vi "load_manual.vi"(8 "error in (no error)":errorcluster) -> (0 "error out":errorcluster, 2 "replaced_action(s)":bool, 3 "manual_actions out":variant)   [LabVIEW 2015, in "lv-recipe-machine.lvlib" / "example_01.lvlib"]
doc: "load_manual.vi will assign manual steps as variant attributes to an empty variant. An indicator is provided if actions are replaced (e.g. a duplicate key)."
uses:
  example_01.lvlib
  public/_controls/step.ctl
  public/_controls/vi_reference_type.ctl
  _controls/steps_actions.ctl
  public/_controls/vi_reference_manual_action.ctl
  lv-recipe-machine.lvlib
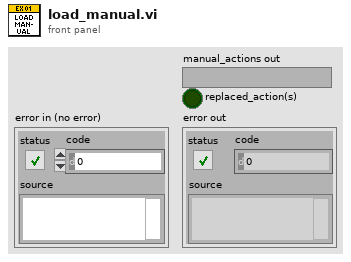
[diagram p1: front panel]
types:
  T1 = typedef "lv-recipe-machine.lvlib/vi_reference_manual_action.ctl" = refnum<vi>
  T2 = typedef "lv-recipe-machine.lvlib/example_01.lvlib/steps_actions.ctl" = enum16{"<steps_actions>", "manual_random", "manual_comparison", "manual_wait", "auto_random", "auto_wait", "criteria_initialize", "criteria_count", "criteria_comparison", "transition_simple", "transition_count", "transition_comparison", "launch_wait", "<null>"}
  T3 = typedef "lv-recipe-machine.lvlib/vi_reference_type.ctl" = enum16{"<vi_reference_type>", "manual_action", "auto_step", "auto_criteria", "auto_transition", "auto_launcher", "<null>"}
  T4 = typedef "lv-recipe-machine.lvlib/step.ctl" = cluster{"name":string, "vi_reference":variant}
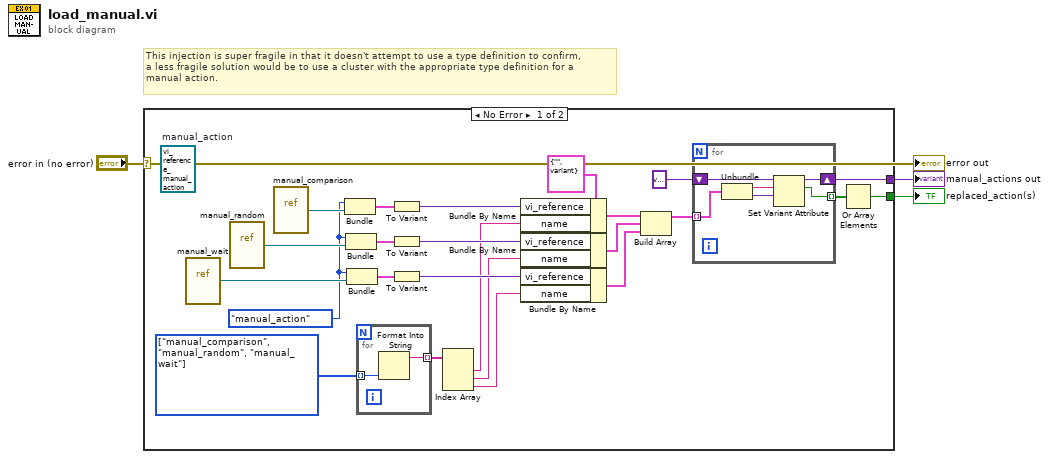
[diagram p0: block diagram]
diagram:
  # "This injection is super fragile in that it doesn't attempt to use a type definition to confirm,\na less fragile solution would be to use a cluster with the appropriate type definition for a\nmanual action."
  n1 = case shown="No Error" "error in (no error)" {
    tunnel: [w25 _] -> w3
    tunnel: [w20 _] -> w2
    frame No Error {
      (unwired) T1 refnum  # manual_action
      w8 = T2[] [enum."manual_comparison", enum."manual_random", enum."manual_wait"] items=["<steps_actions>", "manual_random", "manual_comparison", "manual_wait", "auto_random", "auto_wait", "criteria_initialize", "criteria_count", "criteria_comparison", "transition_simple", "transition_count", "transition_comparison", "launch_wait", "<null>"]
      w9 = vi_reference_type."manual_action" ("vi_reference_type")
      w26 = T4 {"name"="", "vi_reference"=variant(refnum<vi> refnum)} ("step")
      n2 = vi-ref "manual_wait.vi"() -> (w15:refnum<vi>)
      n3 = vi-ref "manual_random.vi"() -> (w13:refnum<vi>)
      n4 = vi-ref "manual_comparison.vi"() -> (w11:refnum<vi>)
      n5 = Bundle("vi_reference_type"=w9, w11) -> (w10:cluster{"vi_reference_type":T3, refnum<vi>})  [unwired: 1 in]
      n6 = Bundle("vi_reference_type"=w9, w13) -> (w12:cluster{"vi_reference_type":T3, refnum<vi>})  [unwired: 1 in]
      n7 = Bundle("vi_reference_type"=w9, w15) -> (w14:cluster{"vi_reference_type":T3, refnum<vi>})  [unwired: 1 in]
      n8 = for {
        tunnel: w8 -> [w29] mode=indexing
        tunnel: [w28] -> w7 mode=indexing
        n9 = Format Into String(w29) -> (resulting string=w28:string)  [unwired: 3 in, 1 out]
      }
      n10 = To Variant(anything=w10) -> (Variant=w18:variant)
      n11 = To Variant(anything=w12) -> (Variant=w17:variant)
      n12 = To Variant(anything=w14) -> (Variant=w16:variant)
      n13 = Index Array(array=w7) -> (element #1=w6:string, element #2=w5:string, element #3=w4:string)  [unwired: 3 in]
      n14 = Bundle By Name(cluster=w26, "vi_reference"=w18, "name"=w6) -> (w22:T4)
      n15 = Bundle By Name(cluster=w26, "vi_reference"=w17, "name"=w5) -> (w23:T4)
      n16 = Bundle By Name(cluster=w26, "vi_reference"=w16, "name"=w4) -> (w27:T4)
      n17 = Build Array(w22, w23, w27) -> (w24:T4[])
      n18 = for {
        tunnel: w24 -> [w33] mode=indexing
        shift-right: [w34] -> w25
        shift-left: variant ("manual_actions in") -> [w35]
        tunnel: [w31] -> w19 mode=indexing
        n19 = Unbundle(w33) -> ("name"=w32:string, "vi_reference"=w30:variant)
        n20 = Set Variant Attribute(Variant=w35, name=w32, value=w30) -> (Variant out=w34:variant, replaced=w31:bool)  [unwired: 1 in, 1 out]
      }
      n21 = Or Array Elements(Boolean array=w19) -> (logical OR=w20:bool)
    }
    frame Error {
    }
  }
  "manual_actions out" <- w3
  "replaced_action(s)" <- w2
  "error out" <- "error in (no error)"
